vi "Destroy.vi"(11 "eeeee in":refnum<class "eeeee.lvclass">) -> (3 "eeeee out":refnum<class "eeeee.lvclass">)   [LabVIEW 2021, in "Providers.lvlib" / "eeeee.lvlib" / "eeeee.lvclass"]
uses:
  eeeee.lvclass
  eeeee.lvclass/eeeee.ctl
  jettl/Event/Event.lvclass
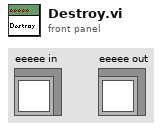
[diagram p1: front panel]
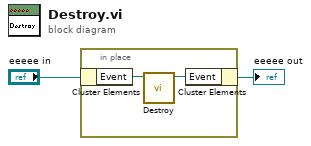
[diagram p0: block diagram]
diagram:
  n1 = in-place {
    n2 = in-place-cluster #1("eeeee in") -> ("Event"=w4:refnum<class "Event.lvclass">)
    n3 = call-dynamic "Destroy.vi"("jettl in"=w4) -> ("jettl out"=w3:refnum<class "Event.lvclass">)  [unwired: 10 in]
    n4 = in-place-cluster #1("Event"=w3) -> (→"eeeee out":refnum<class "eeeee.lvclass">)
  }
